vi "KE6221 -- Get Wave No Trig In Inactive Val.vi"(0 "Resource In":refnum<visa-resource-name>, 1 "Check For SCPI Errors? (T)":bool=TRUE, 11 "error in (no error)":errorcluster) -> (4 "Resource Out (dupl)":refnum<visa-resource-name>, 8 "Inactive Level (%)":T1=50.0 caption="Note:  100% = max, -100% = min" min=-100.0 max=100.0 format="%.3p", 15 "error out":errorcluster)   [LabVIEW 2018, in "Keithley 622x.lvlib"]
uses:
  Keithley 622x.lvlib
  Typedefs/KE6221 -- Wave Inactive Level.ctl
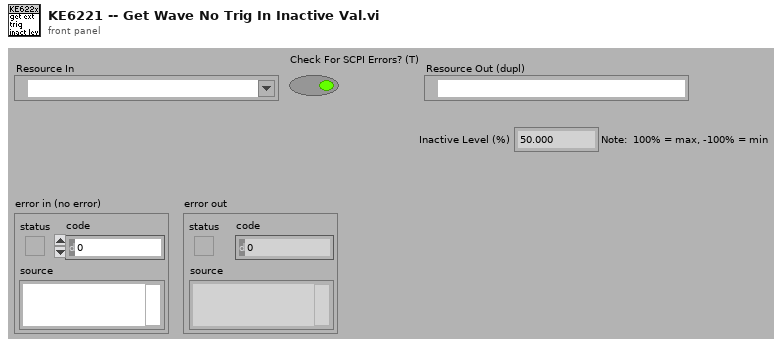
[diagram p1: front panel]
types:
  T1 = typedef "Keithley 622x.lvlib/KE6221 -- Wave Inactive Level.ctl" = dbl
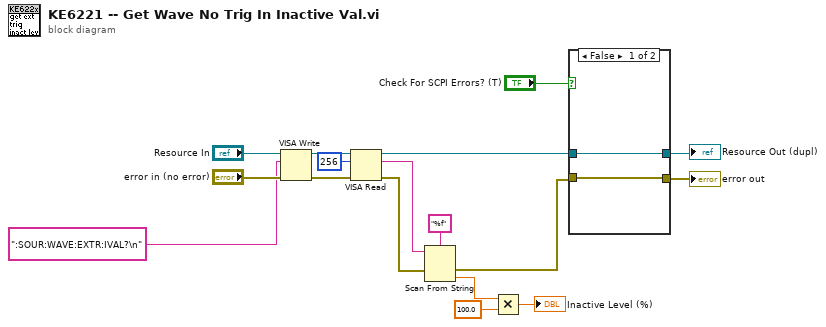
[diagram p0: block diagram]
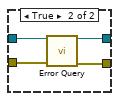
[diagram p2: hidden frame]
diagram:
  n1 = VISA Write(VISA resource name="Resource In", write buffer=":SOUR:WAVE:EXTR:IVAL?\n" ("format string"), error in (no error)="error in (no error)") -> (VISA resource name out=w11:refnum<visa-resource-name>, error out=w10:errorcluster)  [unwired: 1 out]
  n2 = VISA Read(VISA resource name=w11, byte count=u32 256, error in (no error)=w10) -> (VISA resource name out=w4:refnum<visa-resource-name>, read buffer=w6:string, error out=w8:errorcluster)  [unwired: 1 out]
  n3 = Scan From String(format string="%f", input string=w6, error in=w8) -> (error out=w5:errorcluster, output 1=w3:dbl)  [unwired: 2 in, 2 out]
  n4 = Multiply(x=w3, y=100.0) -> (x*y=→"Inactive Level (%)":dbl)
  n5 = case shown="False" "Check For SCPI Errors? (T)" {
    tunnel: w4 -> [w19 w23]
    tunnel: w5 -> [w18 w22]
    tunnel: [w18 w21] -> w13
    tunnel: [w19 w20] -> w14
    frame False {
    }
    frame True {
      n6 = call "Error Query.vi"("VISA Resource In"=w23, "error in (no error)"=w22) -> ("VISA Resource Out (dupl)"=w20:refnum<visa-resource-name>, "error out"=w21:errorcluster)  [unwired: 10 in, 2 out]
    }
  }
  "Resource Out (dupl)" <- w14
  "error out" <- w13
